vi "Y_H_change_state.vi"(8 "error in (no error)":errorcluster, 11 "Y_H_in":refnum<class "Y_H.lvclass">) -> (0 "error out":errorcluster, 3 "Y_H_out":refnum<class "Y_H.lvclass">)   [LabVIEW 2019, in "Y_H.lvclass"]
uses:
  Y_H.lvclass
  Y_H.lvclass/Y_H.ctl
panel:
  in  "setpoint":T1(slide) caption="oC" scale=0.0..500.0 scale format="%#_5g"
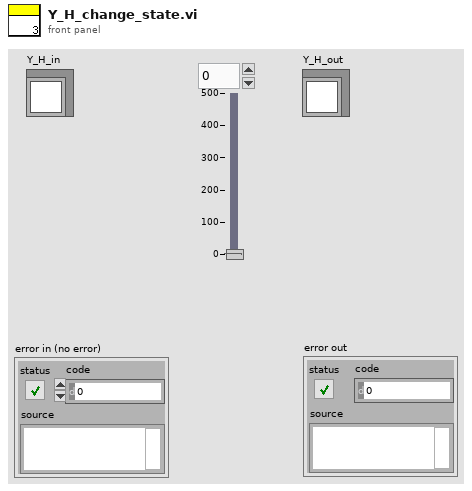
[diagram p1: front panel]
types:
  T1 = cluster{"Numeric":dbl, "Numeric":dbl, "Numeric":dbl}
  T2 = typedef "control.lvlib/Y_source.ctl" = enum8{"initialize", "local disabled", "local hand", "hand", "auto", "dist"}
  T3 = enum8{"Enabled", "Disabled", "Disabled and Grayed Out"}
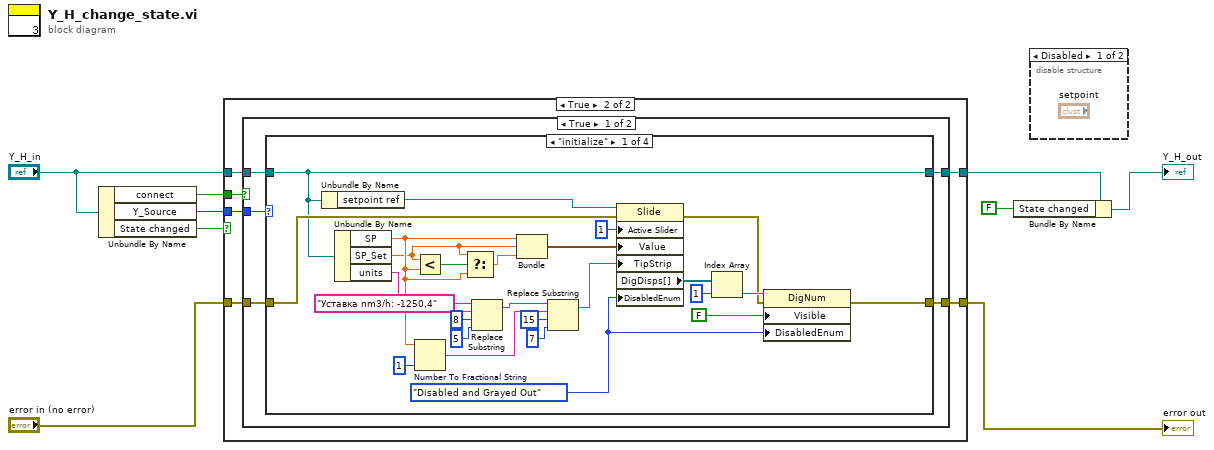
[diagram p0: block diagram]
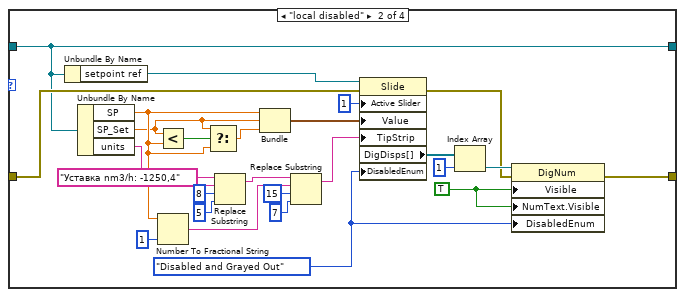
[diagram p3: hidden frame]
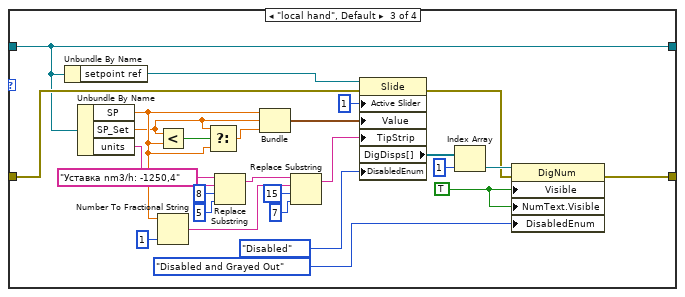
[diagram p4: hidden frame]
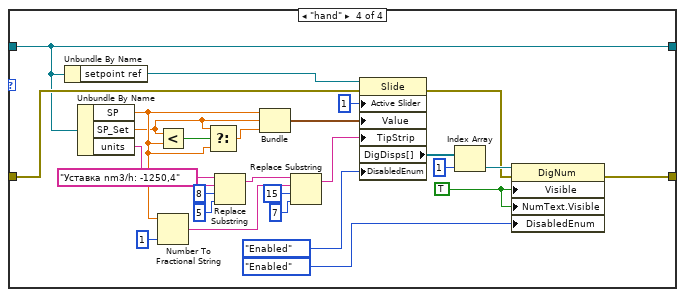
[diagram p5: hidden frame]
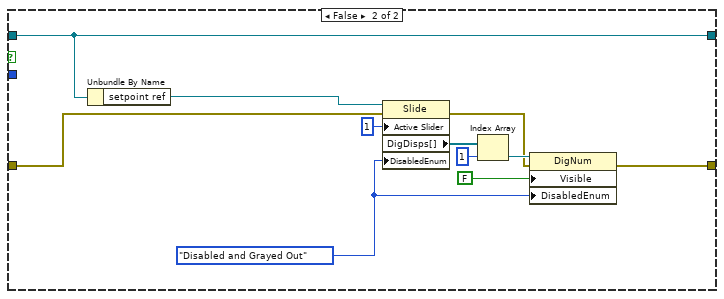
[diagram p6: hidden frame]
diagram:
  n1 = Unbundle By Name("Y_H_in") -> ("connect"=w5:bool, "Y_Source"=w4:T2, "State changed"=w2:bool)
  n2 = case shown="True" w2 {
    tunnel: "error in (no error)" -> [w10 w17]
    tunnel: [w10 w16] -> w7
    tunnel: [w11 w15] -> w1
    tunnel: w5 -> [_ w14]
    tunnel: "Y_H_in" -> [w11 w13]
    tunnel: w4 -> [_ w12]
    frame False {
    }
    frame True {
      n3 = case shown="True" w14 {
        tunnel: w12 -> [w22 _]
        tunnel: [w20 w139] -> w15
        tunnel: w17 -> [w19 w138]
        tunnel: w13 -> [w21 w139]
        tunnel: [w18 w137] -> w16
        frame True {
          n4 = case shown="\"initialize\"" w22 {
            tunnel: w21 -> [w32 w60 w90 w117]
            tunnel: [w32 w60 w90 w117] -> w20
            tunnel: w19 -> [w40 w68 w98 w125]
            tunnel: [w41 w69 w77 w104] -> w18
            frame "initialize" {
              w45 = T3."Disabled and Grayed Out" ("Disabled")
              # "local hand"
              n5 = Unbundle By Name(w32) -> ("setpoint ref"=w43:refnum<vi>)
              n6 = Unbundle By Name(w32) -> ("SP"=w31:dbl, "SP_Set"=w30:dbl, "units"=w24:string)
              n7 = Less?(x=w30, y=w31) -> (x < y?=w38:bool)
              n8 = Number To Fractional String(number=w31, precision (6)=i16 1) -> (F-format string=w25:string)  [unwired: 2 in]
              n9 = Select(t=w30, s=w38, f=w31) -> (s? t:f=w37:dbl)
              n10 = Replace Substring(2:5 ("length (len. of substring)"), 3:8 ("offset (0)"), 4:w24, 5:"Уставка nm3/h: -1250,4") -> (1:w26:string)  [unwired: 1 out]
              n11 = Bundle("SP"=w31, "SP_Set"=w30, "SP"=w37) -> (w29:cluster{"SP":dbl, "SP_Set":dbl, "SP":dbl})  [unwired: 1 in]
              n12 = Replace Substring(2:7 ("length (len. of substring)"), 3:15 ("offset (0)"), 4:w25, 5:w26) -> (1:w23:string)  [unwired: 1 out]
              n13 = property on="Property Node" class="Slide"(reference=w43, error in=w40, "Active Slider"=1, "Value"=w29, "TipStrip"=w23, "DisabledEnum"=w45) -> (error out=w42:errorcluster, "DigDisps[]"=w44:refnum<vi>[])  [unwired: 1 out]
              n14 = Index Array(array=w44, index=1) -> (element=w48:refnum<vi>)
              n15 = property class="DigNum"(reference=w48, error in=w42, "Visible"=FALSE ("Z_ASwitch"), "DisabledEnum"=w45) -> (error out=w41:errorcluster)  [unwired: 1 out]
            }
            frame "local disabled" {
              w49 = TRUE ("Z_ASwitch")
              w50 = T3."Disabled and Grayed Out" ("Disabled")
              # "local hand"
              n16 = Unbundle By Name(w60) -> ("setpoint ref"=w71:refnum<vi>)
              n17 = Unbundle By Name(w60) -> ("SP"=w59:dbl, "SP_Set"=w58:dbl, "units"=w52:string)
              n18 = Less?(x=w58, y=w59) -> (x < y?=w66:bool)
              n19 = Number To Fractional String(number=w59, precision (6)=i16 1) -> (F-format string=w53:string)  [unwired: 2 in]
              n20 = Select(t=w58, s=w66, f=w59) -> (s? t:f=w65:dbl)
              n21 = Replace Substring(2:5 ("length (len. of substring)"), 3:8 ("offset (0)"), 4:w52, 5:"Уставка nm3/h: -1250,4") -> (1:w54:string)  [unwired: 1 out]
              n22 = Bundle("SP"=w59, "SP_Set"=w58, "SP"=w65) -> (w57:cluster{"SP":dbl, "SP_Set":dbl, "SP":dbl})  [unwired: 1 in]
              n23 = Replace Substring(2:7 ("length (len. of substring)"), 3:15 ("offset (0)"), 4:w53, 5:w54) -> (1:w51:string)  [unwired: 1 out]
              n24 = property on="Property Node" class="Slide"(reference=w71, error in=w68, "Active Slider"=1, "Value"=w57, "TipStrip"=w51, "DisabledEnum"=w50) -> (error out=w70:errorcluster, "DigDisps[]"=w72:refnum<vi>[])  [unwired: 1 out]
              n25 = Index Array(array=w72, index=1) -> (element=w74:refnum<vi>)
              n26 = property class="DigNum"(reference=w74, error in=w70, "Visible"=w49, "NumText.Visible"=w49, "DisabledEnum"=w50) -> (error out=w69:errorcluster)  [unwired: 1 out]
            }
            frame "local hand", Default {
              w75 = TRUE ("Z_ASwitch")
              # "local hand"
              n27 = Unbundle By Name(w90) -> ("setpoint ref"=w99:refnum<vi>)
              n28 = Unbundle By Name(w90) -> ("SP"=w89:dbl, "SP_Set"=w88:dbl, "units"=w82:string)
              n29 = Less?(x=w88, y=w89) -> (x < y?=w96:bool)
              n30 = Number To Fractional String(number=w89, precision (6)=i16 1) -> (F-format string=w83:string)  [unwired: 2 in]
              n31 = Select(t=w88, s=w96, f=w89) -> (s? t:f=w95:dbl)
              n32 = Replace Substring(2:5 ("length (len. of substring)"), 3:8 ("offset (0)"), 4:w82, 5:"Уставка nm3/h: -1250,4") -> (1:w84:string)  [unwired: 1 out]
              n33 = Bundle("SP"=w89, "SP_Set"=w88, "SP"=w95) -> (w87:cluster{"SP":dbl, "SP_Set":dbl, "SP":dbl})  [unwired: 1 in]
              n34 = Replace Substring(2:7 ("length (len. of substring)"), 3:15 ("offset (0)"), 4:w83, 5:w84) -> (1:w81:string)  [unwired: 1 out]
              n35 = property on="Property Node" class="Slide"(reference=w99, error in=w98, "Active Slider"=1, "Value"=w87, "TipStrip"=w81, "DisabledEnum"=T3."Disabled" ("Disabled")) -> (error out=w78:errorcluster, "DigDisps[]"=w100:refnum<vi>[])  [unwired: 1 out]
              n36 = Index Array(array=w100, index=1) -> (element=w79:refnum<vi>)
              n37 = property class="DigNum"(reference=w79, error in=w78, "Visible"=w75, "NumText.Visible"=w75, "DisabledEnum"=T3."Disabled and Grayed Out" ("Disabled")) -> (error out=w77:errorcluster)  [unwired: 1 out]
            }
            frame "hand" {
              w102 = TRUE ("Z_ASwitch")
              # "local hand"
              n38 = Unbundle By Name(w117) -> ("setpoint ref"=w126:refnum<vi>)
              n39 = Unbundle By Name(w117) -> ("SP"=w116:dbl, "SP_Set"=w115:dbl, "units"=w109:string)
              n40 = Less?(x=w115, y=w116) -> (x < y?=w123:bool)
              n41 = Number To Fractional String(number=w116, precision (6)=i16 1) -> (F-format string=w110:string)  [unwired: 2 in]
              n42 = Select(t=w115, s=w123, f=w116) -> (s? t:f=w122:dbl)
              n43 = Replace Substring(2:5 ("length (len. of substring)"), 3:8 ("offset (0)"), 4:w109, 5:"Уставка nm3/h: -1250,4") -> (1:w111:string)  [unwired: 1 out]
              n44 = Bundle("SP"=w116, "SP_Set"=w115, "SP"=w122) -> (w114:cluster{"SP":dbl, "SP_Set":dbl, "SP":dbl})  [unwired: 1 in]
              n45 = Replace Substring(2:7 ("length (len. of substring)"), 3:15 ("offset (0)"), 4:w110, 5:w111) -> (1:w108:string)  [unwired: 1 out]
              n46 = property on="Property Node" class="Slide"(reference=w126, error in=w125, "Active Slider"=1, "Value"=w114, "TipStrip"=w108, "DisabledEnum"=T3."Enabled" ("Disabled")) -> (error out=w105:errorcluster, "DigDisps[]"=w127:refnum<vi>[])  [unwired: 1 out]
              n47 = Index Array(array=w127, index=1) -> (element=w106:refnum<vi>)
              n48 = property class="DigNum"(reference=w106, error in=w105, "Visible"=w102, "NumText.Visible"=w102, "DisabledEnum"=T3."Enabled" ("Disabled")) -> (error out=w104:errorcluster)  [unwired: 1 out]
            }
          }
        }
        frame False {
          w133 = T3."Disabled and Grayed Out" ("Disabled")
          n49 = Unbundle By Name(w139) -> ("setpoint ref"=w131:refnum<vi>)
          n50 = property on="Property Node" class="Slide"(reference=w131, error in=w138, "Active Slider"=1, "DisabledEnum"=w133) -> (error out=w130:errorcluster, "DigDisps[]"=w132:refnum<vi>[])  [unwired: 1 out]
          n51 = Index Array(array=w132, index=1) -> (element=w136:refnum<vi>)
          n52 = property class="DigNum"(reference=w136, error in=w130, "Visible"=FALSE ("Z_ASwitch"), "DisabledEnum"=w133) -> (error out=w137:errorcluster)  [unwired: 1 out]
        }
      }
    }
  }
  "error out" <- w7
  n53 = Bundle By Name(cluster=w1, "State changed"=FALSE ("Data changed")) -> (→"Y_H_out":refnum<class "Y_H.lvclass">)
  n54 = disable-structure shown="Disabled" {
    frame Disabled {
    }
    frame Enabled {
    }
  }
